vi "Get Wait Until Data.vi"(8 "error in (no error)":errorcluster, 11 "Queue in":refnum<queue>) -> (0 "error out":errorcluster, 2 "Data":dbl)   [LabVIEW 2018, in "Sequencing Library.lvlib"]
uses:
  Sequencing Library.lvlib
  support/Message Queue/Message Cluster.ctl
  support/Message Queue/Enqueue Message (Single).vi
  support/Message Queue/Message Queue.lvlib
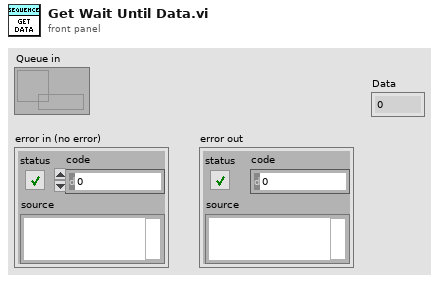
[diagram p1: front panel]
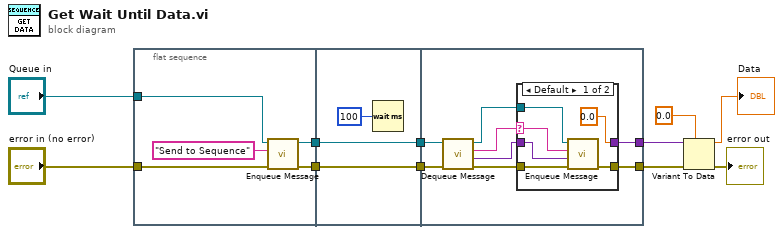
[diagram p0: block diagram]
diagram:
  n1 = flat-sequence {
    tunnel: "Queue in" -> [w16]
    tunnel: "error in (no error)" -> [w15]
    tunnel: [w13] -> w11
    tunnel: [w12] -> w10
    tunnel: [w19] -> w9
    tunnel: w11 -> [w19]
    tunnel: [w18] -> w8
    tunnel: w10 -> [w18]
    tunnel: [w20] -> w2
    tunnel: w9 -> [w27]
    tunnel: w8 -> [w26]
    tunnel: [w24] -> w5
    frame #0 {
      n2 = call-poly "Enqueue Message.vi"("error in (no error)"=w15, "Message"="Send to Sequence", "Message Queue"=w16) -> ("error out"=w13:errorcluster, "dup Message Queue"=w12:refnum<queue>)  [unwired: 7 in]
    }
    frame #1 {
      n3 = Wait (ms)(milliseconds to wait=u32 100) -> ()  [unwired: 1 out]
    }
    frame #2 {
      n4 = call "Dequeue Message.vi"("error in (no error)"=w27, "Message Queue"=w26) -> ("error out"=w21:errorcluster, "Message Data"=w23:variant, "Message"=w25:string, "dup Message Queue"=w22:refnum<queue>)  [unwired: 6 in]
      n5 = case shown="Default" w25 {
        selector: w25 -> [w33 _]
        tunnel: [0.0 w35] -> w24
        tunnel: w23 -> [w32 w35]
        tunnel: w22 -> [w31 _]
        tunnel: w21 -> [w30 w34]
        tunnel: [w29 w34] -> w20
        frame Default {
          n6 = call-poly "Enqueue Message.vi"("error in (no error)"=w30, "Message Data"=w32, "Message"=w33, "Message Queue"=w31) -> ("error out"=w29:errorcluster)  [unwired: 6 in, 1 out]
        }
        frame "Sent to Sequence" {
        }
      }
    }
  }
  n7 = Variant To Data(error in=w2, type=0.0, Variant=w5) -> (data=→"Data":dbl, error out=→"error out":errorcluster)
